vi "onUnhandledDependencyError.vi"(7 "Stop on Unhandled Error (F)":bool, 8 "Unhandled Dependency Error":errorcluster, 9 "Dependency":refnum<class "SMO.lvclass">, 11 "SMO.ErrorInjection in":refnum<class "SMO.ErrorInjection.lvclass">) -> (0 "Unhandled error":errorcluster, 3 "SMO.ErrorInjection out":refnum<class "SMO.ErrorInjection.lvclass">)   [LabVIEW 2021, in "SMO.ErrorInjection.lvclass"]
uses:
  SMO.ErrorInjection.lvclass
  SMO.ErrorInjection.lvclass/SMO.ErrorInjection.ctl
  src/SMO/SMO.lvclass
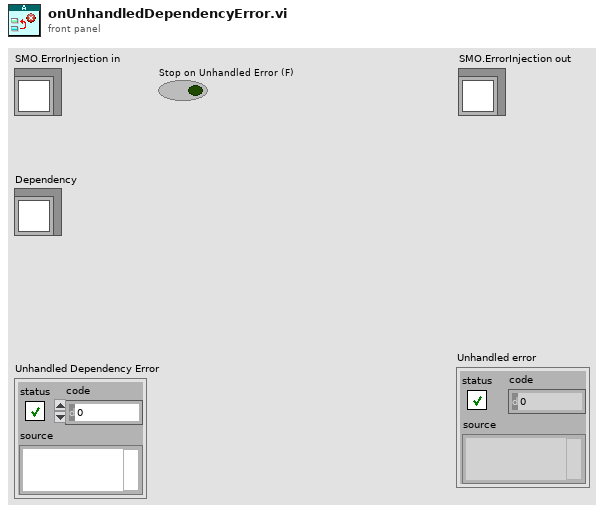
[diagram p1: front panel]
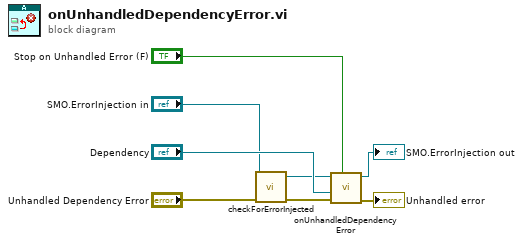
[diagram p0: block diagram]
diagram:
  n1 = call "checkForErrorInjected.vi"("error in (no error)"="Unhandled Dependency Error", "SMO.ErrorInjection in"="SMO.ErrorInjection in") -> ("error out"=w3:errorcluster, "SMO.ErrorInjection dup"=w2:refnum<class "SMO.ErrorInjection.lvclass">)  [unwired: 8 in]
  n2 = call-parent "onUnhandledDependencyError.vi"("(deprecated -- use Handle Error override)"="Stop on Unhandled Error (F)", "Unhandled Dependency Error"=w3, "Dependency"="Dependency", "SMO in"=w2) -> ("Unhandled error"=→"Unhandled error":errorcluster, "SMO out"=→"SMO.ErrorInjection out":refnum<class "SMO.ErrorInjection.lvclass">)  [unwired: 6 in]
